vi "SendCalibrationsToDB.vi"   [LabVIEW 2016]
uses:
  Configurations.vi
  <vilib>/Rock Robotics/Network Tables/NT Write Numeric Array.vi
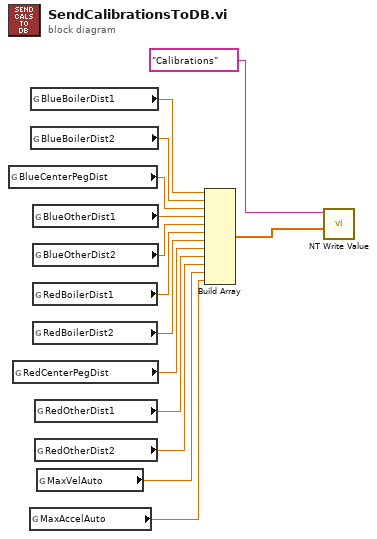
[diagram p0: block diagram]
diagram:
  n1 = global read "Configurations.vi" "BlueCenterPegDist"() -> (w11:dbl)
  n2 = global read "Configurations.vi" "RedCenterPegDist"() -> (w6:dbl)
  n3 = global read "Configurations.vi" "MaxAccelAuto"() -> (w1:dbl)
  n4 = global read "Configurations.vi" "BlueBoilerDist1"() -> (w13:dbl)
  n5 = global read "Configurations.vi" "BlueBoilerDist2"() -> (w12:dbl)
  n6 = global read "Configurations.vi" "BlueOtherDist1"() -> (w10:dbl)
  n7 = global read "Configurations.vi" "BlueOtherDist2"() -> (w9:dbl)
  n8 = global read "Configurations.vi" "RedBoilerDist1"() -> (w8:dbl)
  n9 = global read "Configurations.vi" "RedBoilerDist2"() -> (w7:dbl)
  n10 = global read "Configurations.vi" "RedOtherDist1"() -> (w5:dbl)
  n11 = global read "Configurations.vi" "RedOtherDist2"() -> (w4:dbl)
  n12 = global read "Configurations.vi" "MaxVelAuto"() -> (w2:dbl)
  n13 = Build Array(w13, w12, w11, w10, w9, w8, w7, w6, w5, w4, w2, w1) -> (w3:dbl[])
  n14 = call-poly <vilib>:"NT Write Value.vi"("Numeric Array"=w3, "Name"="Calibrations") -> ()  [unwired: 9 in, 1 out]
